vi "Pack Launch Nested Views Msg.vi"(10 "View Labels":string[](array[string]), 11 "Nested Views":refnum<class "IViewable.lvclass">[](array[class])) -> (3 "Launch Nested Views Msg":refnum<class "Launch Nested Views Msg.lvclass">)   [LabVIEW 2020, in "IViewManager.lvlib" / "Launch Nested Views Msg.lvclass"]
doc: "包装启动嵌套视图消息"
uses:
  Launch Nested Views Msg.lvclass
  IViewable/IViewable/IViewable.lvclass
  Launch Nested Views Msg.lvclass/Launch Nested Views Msg.ctl
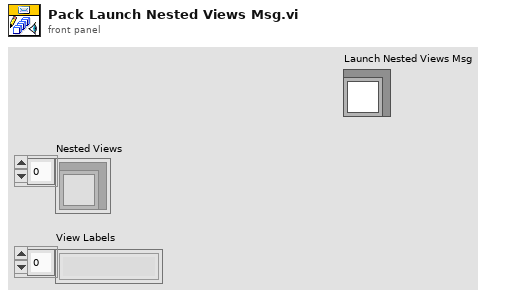
[diagram p1: front panel]
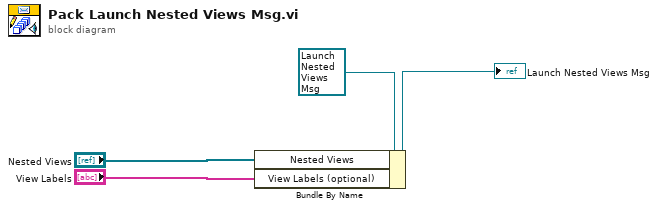
[diagram p0: block diagram]
diagram:
  n1 = Bundle By Name(cluster=refnum<class "Launch Nested Views Msg.lvclass"> refnum ("Launch Nested Views Msg in"), "Nested Views"="Nested Views", "View Labels (optional)"="View Labels") -> (→"Launch Nested Views Msg":refnum<class "Launch Nested Views Msg.lvclass">)
